vi "Clear Errors.vi"(4 "error in (no error)":errorcluster, 7 "specific error code to clear (0: all)":i32) -> (0 "error out":errorcluster, 3 "specific error cleared?":bool)   [LabVIEW 2015]
doc: "Resets the error <B>status</B> to no error, <B>code</B> to 0, and <B>source</B> to an empty string. Use this VI when you want to ignore an error. By default, this VI ignores all errors. Wire an error code value to <B>specific error code to clear</B> if you only want to ignore a specific error."
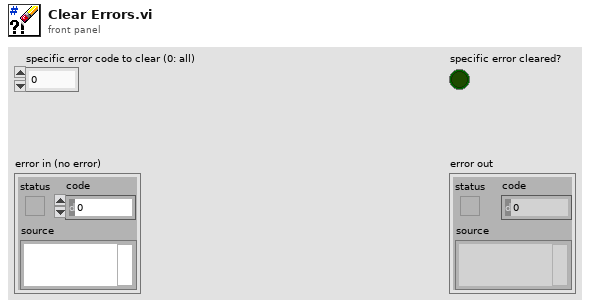
[diagram p1: front panel]
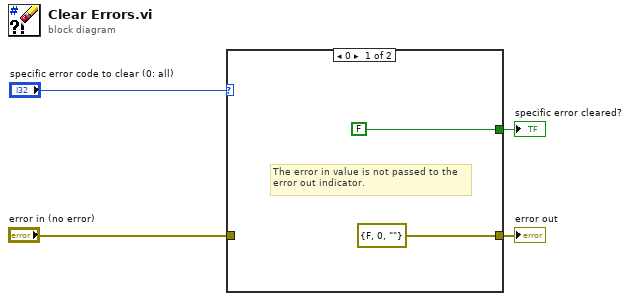
[diagram p0: block diagram]
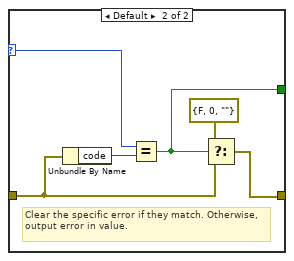
[diagram p2: hidden frame]
diagram:
  n1 = case shown="0" "specific error code to clear (0: all)" {
    selector: "specific error code to clear (0: all)" -> [_ w11]
    tunnel: "error in (no error)" -> [_ w10]
    tunnel: [errorcluster {"status"=FALSE, "code"=0, "source"=""} ("error constant") w7] -> w2
    tunnel: [FALSE w8] -> w1
    frame 0 {
      # "The error in value is not passed to the\nerror out indicator."
    }
    frame Default {
      # "Clear the specific error if they match. Otherwise, output error in value."
      n2 = Unbundle By Name(w10) -> ("code"=w12:i32)
      n3 = Equal?(x=w11, y=w12) -> (x = y?=w8:bool)
      n4 = Select(t=errorcluster {"status"=FALSE, "code"=0, "source"=""} ("error constant"), s=w8, f=w10) -> (s? t:f=w7:errorcluster)
    }
  }
  "error out" <- w2
  "specific error cleared?" <- w1
